vi "AudioTest.Load Plot Limit Definitions From Config File.vi"(8 "error in (no error)":errorcluster, 11 "Config Folder":path=path "C:/MTE/Audio Test/Config") -> (0 "error out":errorcluster, 3 "LimitPlots":T1[](array[typedef]))   [LabVIEW 2018]
uses:
  TypeDefs/AudioTest.Result Plot Data.ctl
  Common/Utils/Errors/Error.Error Code List.ctl
  <vilib>/KATE/Files/File Utils.lvlib
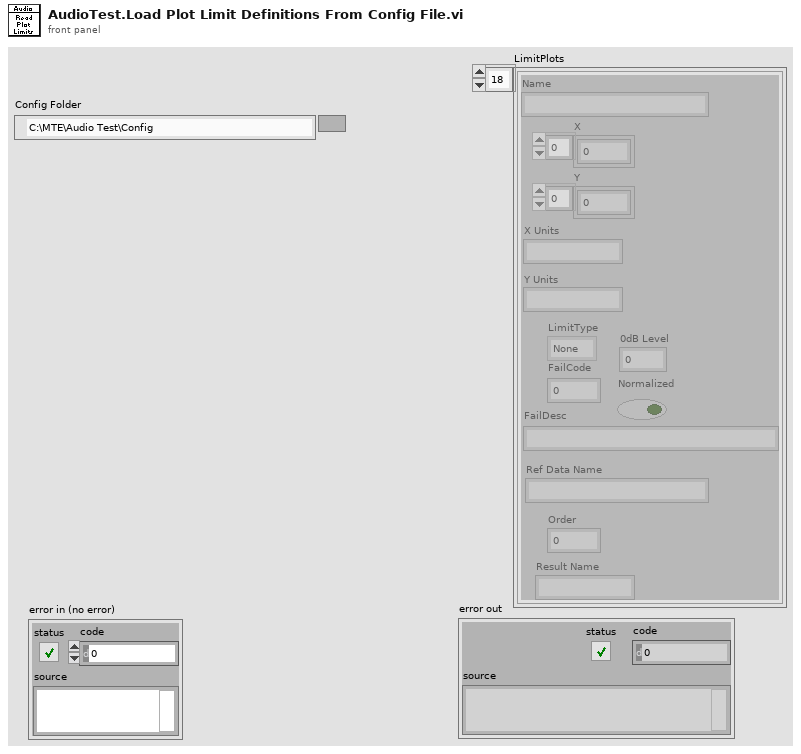
[diagram p1: front panel]
types:
  T1 = typedef "AudioTest.Result Plot Data.ctl" = cluster{"Order":i32, "Name":string, "X":dbl[], "Y":dbl[], "X Units":string, "Y Units":string, "LimitType":enum16{"None", "LL", "UL"}, "FailCode":i32, "FailDesc":string, "Ref Data Name":string, "Result Name":string, "0dB Level":dbl, "Normalized":bool}
  T2 = typedef "Error.Error Code List.ctl" = i32
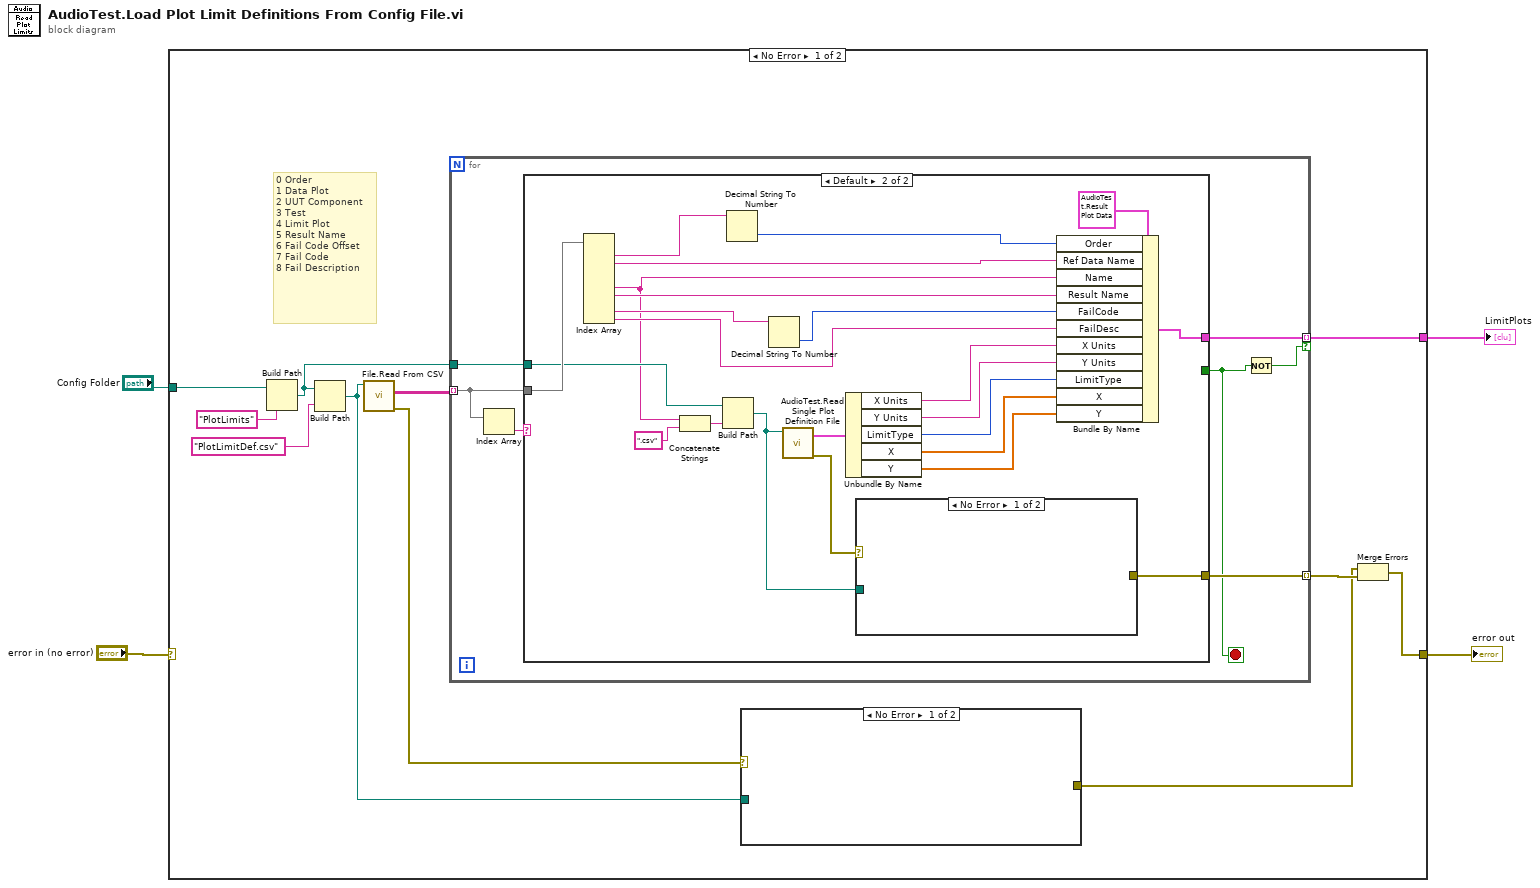
[diagram p0: block diagram]
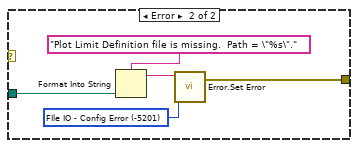
[diagram p2: hidden frame]
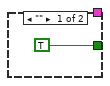
[diagram p3: hidden frame]
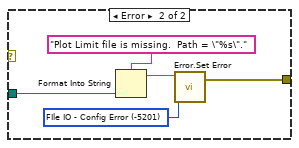
[diagram p4: hidden frame]
diagram:
  n1 = case shown="No Error" "error in (no error)" {
    selector: "error in (no error)" -> [_ w57]
    tunnel: "Config Folder" -> [w15 _]
    tunnel: [w13 _] -> w3
    tunnel: [w8 w57] -> w1
    frame No Error {
      # "0 Order\n1 Data Plot\n2 UUT Component\n3 Test\n4 Limit Plot\n5 Result Name\n6 Fail Code Offset\n7 Fail Code\n8 Fail Description"
      n2 = Build Path(base path=w15, name or relative path="PlotLimits") -> (appended path=w10:path)
      n3 = Build Path(base path=w10, name or relative path="PlotLimitDef.csv") -> (appended path=w6:path)
      n4 = call <vilib>:"File.Read From CSV.vi"("File"=w6) -> ("error out"=w7:errorcluster, "Data"=w11:string[][])  [unwired: 8 in, 1 out]
      n5 = for {
        tunnel: w11 -> [w24] mode=indexing
        tunnel: [w26] -> w13 mode=indexing if=w22
        tunnel: w10 -> [w27]
        tunnel: [w25] -> w9 mode=indexing
        stop <- w21 stop-if-true
        n6 = Index Array(array=w24) -> (element=w23:string)  [unwired: 1 in]
        n7 = case shown="Default" w23 {
          tunnel: w24 -> [_ w50]
          tunnel: w27 -> [_ w40]
          tunnel: [_ w33] -> w26
          tunnel: [_ w30] -> w25
          tunnel: [TRUE _] -> w21
          frame "" {
          }
          frame Default {
            n8 = Index Array(array=w50) -> (element #1=w49:string, element #2=w47:string, element #5=w29:string, element #6=w46:string, element #8=w45:string, element #9=w43:string)  [unwired: 9 in, 3 out]
            n9 = Concatenate Strings(w29, ".csv" ("string")) -> (w42:string)
            n10 = Build Path(base path=w40, name or relative path=w42) -> (appended path=w31:path)
            n11 = Decimal String To Number(string=w49) -> (number=w48:i32)  [unwired: 2 in, 1 out]
            n12 = Decimal String To Number(string=w45) -> (number=w44:i32)  [unwired: 2 in, 1 out]
            n13 = call "AudioTest.Read Single Plot Definition File.vi"("CSV File"=w31) -> ("error out"=w32:errorcluster, "Plot"=w39:T1)  [unwired: 9 in]
            n14 = Unbundle By Name(w39) -> ("X Units"=w38:string, "Y Units"=w37:string, "LimitType"=w36:enum16{"None", "LL", "UL"}, "X"=w35:dbl[], "Y"=w34:dbl[])
            n15 = case shown="No Error" w32 {
              tunnel: w31 -> [_ w54]
              tunnel: [_ w53] -> w30
              frame No Error {
              }
              frame Error {
                w52 = T2 -5201 items=["No Error"=0, "Abort"=-2, "Misc"=-5000, "Fixture Error"=-5100, "File IO - General"=-5200, "FIle IO - Config Error"=-5201, "Instrument - General"=-5300, "Instrument - Serial Com"=-5301, "Instrument - Camera"=-5302, "Instrument - PS"=-5303, "Instrument - Oscilloscope"=-5304, "Instrument - Function Gen"=-5305, "Instrument - Load"=-5306, "Instrument - Meter"=-5307, "Instrument - Power Control"=-5308, "Instrument - Motion"=-5309, "Instrument - RF"=-5310, "System Exe"=-5400, "Image Processing"=-5500, "Communication"=-5600, "Script - Syntax Error"=-6000, "Script - Invalid Name or Param"=-6100, "Script - Timeout"=-6200, "Invalid Data"=-6300, "FW Update Error"=-6500] ("Std Code")
                n16 = Format Into String(format string="Plot Limit file is missing.  Path = \"%s\".", w54) -> (resulting string=w56:string)  [unwired: 2 in, 1 out]
                n17 = call "Error.Set Error.vi"("Code"=w52, "Desc"=w56) -> ("error out"=w53:errorcluster)  [unwired: 5 in]
              }
            }
            n18 = Bundle By Name(cluster=T1 {"Order"=0, "Name"="", "X"=[], "Y"=[], "X Units"="", "Y Units"="", "LimitType"=enum."None", "FailCode"=0, "FailDesc"="", "Ref Data Name"="", "Result Name"="", "0dB Level"=0.0, "Normalized"=FALSE}, "Order"=w48, "Ref Data Name"=w47, "Name"=w29, "Result Name"=w46, "FailCode"=w44, "FailDesc"=w43, "X Units"=w38, "Y Units"=w37, "LimitType"=w36, "X"=w35, "Y"=w34) -> (w33:T1)
          }
        }
        n19 = Not(x=w21) -> (.not. x?=w22:bool)
      }
      n20 = case shown="No Error" w7 {
        tunnel: w6 -> [_ w18]
        tunnel: [_ w17] -> w5
        frame No Error {
        }
        frame Error {
          w16 = T2 -5201 items=["No Error"=0, "Abort"=-2, "Misc"=-5000, "Fixture Error"=-5100, "File IO - General"=-5200, "FIle IO - Config Error"=-5201, "Instrument - General"=-5300, "Instrument - Serial Com"=-5301, "Instrument - Camera"=-5302, "Instrument - PS"=-5303, "Instrument - Oscilloscope"=-5304, "Instrument - Function Gen"=-5305, "Instrument - Load"=-5306, "Instrument - Meter"=-5307, "Instrument - Power Control"=-5308, "Instrument - Motion"=-5309, "Instrument - RF"=-5310, "System Exe"=-5400, "Image Processing"=-5500, "Communication"=-5600, "Script - Syntax Error"=-6000, "Script - Invalid Name or Param"=-6100, "Script - Timeout"=-6200, "Invalid Data"=-6300, "FW Update Error"=-6500] ("Std Code")
          n21 = Format Into String(format string="Plot Limit Definition file is missing.  Path = \"%s\".", w18) -> (resulting string=w20:string)  [unwired: 2 in, 1 out]
          n22 = call "Error.Set Error.vi"("Code"=w16, "Desc"=w20) -> ("error out"=w17:errorcluster)  [unwired: 5 in]
        }
      }
      n23 = Merge Errors(w5, w9) -> (w8:errorcluster)
    }
    frame Error {
    }
  }
  "LimitPlots" <- w3
  "error out" <- w1
